vi "UHR-Fleezers Control (host) - Lorentz v4.vi"() -> ()   [LabVIEW 2014] (continued)
            n495 = property on="Green Laser ON" class="Bool (strict)"("Val(Sgnl)"=w901) -> ()  [unwired: 2 in, 2 out]
            n496 = property on="Trap Pos. FB ON" class="Bool (strict)"("Val(Sgnl)"=w901) -> ()  [unwired: 2 in, 2 out]
            n497 = property on="Trap Trig. Fl." class="Bool (strict)"("Val(Sgnl)"=w901) -> ()  [unwired: 2 in, 2 out]
            n498 = property on="Fl. Triggered..." class="Bool (strict)"("Val(Sgnl)"=w901) -> ()  [unwired: 2 in, 2 out]
            n499 = property on="Dip for Protein" class="Bool (strict)"("Val(Sgnl)"=w901) -> ()  [unwired: 2 in, 2 out]
            n500 = property on="Pause dwell" class="Bool (strict)"("Val(Sgnl)"=w901) -> ()  [unwired: 2 in, 2 out]
          }
          frame #2 {
            n501 = property on="Trap Pos. FB Offset Factor" class="DigNum (strict)"("Val(Sgnl)"=i64 0 ("Value (Signaling)")) -> ()  [unwired: 2 in, 2 out]
          }
          frame #3 {
            n502 = local read "Saved Stage Positions"() -> (w910:dbl[][])
            n503 = local write "Stage Moving"(TRUE ("Stage Moving")) -> ()
            n504 = Array Subset(array=w910, index (row)=3 ("index"), length (row)=1 ("length"), index (col)=1 ("index"), length (col)=3 ("length")) -> (w915:dbl[][])
            n505 = Reshape Array(w915, 3 ("dimension size")) -> (w913:dbl[])
            n506 = Array To Cluster(array=w913) -> (cluster=w912:cluster{"[0]":dbl, "[1]":dbl, "[2]":dbl})
            n507 = call "Set Stage Position.vi"("Position"=w912, "error in"=w908, "VISA resource name in"=w909) -> ()  [unwired: 3 out]
          }
          frame #4 {
            w920 = FALSE ("Value (Signaling)")
            n508 = case shown="True" w919 {
              frame False {
              }
              frame True {
                n509 = property on="Sample Channel\nFlow" class="Bool (strict)"("Val(Sgnl)"=FALSE ("Stage Moving")) -> ()  [unwired: 2 in, 2 out]
              }
            }
            n510 = property on="Trap 1 (ON/OFF)" class="Bool (strict)"("Val(Sgnl)"=w920) -> ()  [unwired: 2 in, 2 out]
            n511 = property on="Trap 2 (ON/OFF)" class="Bool (strict)"("Val(Sgnl)"=w920) -> ()  [unwired: 2 in, 2 out]
            n512 = call <vilib>:"Beep.vi"() -> ()  [unwired: 3 in, 9 out]
          }
          frame #5 {
            n513 = property on="Move Cap. 2 (ADig Top)" class="Bool (strict)"("Val(Sgnl)"=TRUE ("Value (Signaling)")) -> ()  [unwired: 2 in, 2 out]
            n514 = property on="Tab Control" class="TabCtl (strict)"("Val(Sgnl)"=T51."Status" ("Value (Signaling)")) -> ()  [unwired: 2 in, 2 out]
          }
        }
      }
      event "Dip for Protein": Value Change {
        n515 = event-data() -> ()  [unwired: 1 in, 5 out]
        n516 = case shown="True" "Dip for Protein" {
          tunnel: w926 -> [_ w928]
          tunnel: w925 -> [_ w927]
          frame False {
          }
          frame True {
            n517 = while {
              tunnel: w928 -> [w939]
              tunnel: w927 -> [w938]
              i -> [w933]
              stop <- w935 stop-if-true
              n518 = Increment(x=w933) -> (x+1=→"Dip #":i32)
              n519 = flat-sequence {
                tunnel: w938 -> [w950]
                tunnel: w939 -> [w951]
                tunnel: [w951] -> w943
                tunnel: [w950] -> w942
                tunnel: [w944] -> w929
                tunnel: [w956] -> w937
                tunnel: [w957] -> w936
                tunnel: w943 -> [w958]
                tunnel: w942 -> [w959]
                tunnel: [w954] -> w930
                tunnel: w929 -> [w954]
                tunnel: [w967] -> w941
                tunnel: w937 -> [w967]
                tunnel: [w966] -> w940
                tunnel: w936 -> [w966]
                tunnel: [w963] -> w934
                tunnel: [w962] -> w931
                tunnel: w930 -> [w962]
                tunnel: w940 -> [w987]
                tunnel: w941 -> [w988]
                tunnel: w934 -> [w989]
                tunnel: w931 -> [w986]
                tunnel: [w1045] -> w935
                frame #0 {
                  n520 = local read "Trap Pos. FB ON"() -> (w944:bool)
                  n521 = Compound Arithmetic op=AND("Flow ON\nduring dip?", "FB OFF when \nflow ON", w944) -> (w945:bool)
                  n522 = case shown="True" "Move trap \nbefore dip move?" {
                    frame False {
                    }
                    frame True {
                      n523 = property on="Trap Delta (MHz)" class="DigNum (strict)"("Val(Sgnl)"="Dipping Delta (MHz)") -> ()  [unwired: 2 in, 2 out]
                    }
                  }
                  n524 = property on="Green Laser ON" class="Bool (strict)"("Val(Sgnl)"="Green ON\nbefore dip?") -> ()  [unwired: 2 in, 2 out]
                  n525 = property on="Sample Channel\nFlow" class="Bool (strict)"("Val(Sgnl)"="Flow ON\nduring dip?") -> ()  [unwired: 2 in, 2 out]
                  n526 = case shown="True" w945 {
                    frame False {
                    }
                    frame True {
                      n527 = property on="Trap Pos. FB ON" class="Bool (strict)"("Val(Sgnl)"=FALSE ("Value (Signaling)")) -> ()  [unwired: 2 in, 2 out]
                    }
                  }
                }
                frame #1 {
                  n528 = local read "Saved Stage Positions"() -> (w961:dbl[][])
                  n529 = local write "Cancel dwell"(FALSE ("Cancel dwell")) -> ()
                  n530 = call "move to saved stage position.vi"("error in"=w959, "Stage VISA resource name in"=w958, "Position"="Dip Stage \nPosition", "Saved Stage Positions"=w961) -> ("VISA resource name out"=w956:refnum<visa-resource-name>, "error out"=w957:errorcluster)
                }
                frame #2 {
                  n531 = node-c288() -> (w965:T35)  [unwired: 4 in]
                  n532 = timed-loop {
                    timing: w965 -> [_]
                    timing-out: [_] -> w964
                    tunnel: [w971] -> w963
                    i -> [w968]
                    stop <- w972 stop-if-true
                    n533 = node-c288() -> ()  [unwired: 1 in, 1 out]
                    n534 = Greater Or Equal?(x=w968, y="Dip Duration (s)") -> (x >= y?=w980:bool)
                    n535 = local read "Dip for Protein"() -> (w973:bool)
                    n536 = local read "Dump Beads"() -> (w970:bool)
                    n537 = local read "Cancel dwell"() -> (w979:bool)
                    n538 = local read "Pause dwell"() -> (w976:bool)
                    n539 = Not(x=w973) -> (.not. x?=w978:bool)
                    n540 = Compound Arithmetic op=OR(w979, w980, w978) -> (w977:bool)
                    n541 = Select(t=FALSE, s=w976, f=w977) -> (s? t:f=w974:bool)
                    n542 = Not(x=w970) -> (.not. x?=w969:bool)
                    n543 = node-c288() -> ()  [unwired: 1 in, 1 out]
                    n544 = And(x=w973, y=w969) -> (x .and. y?=w971:bool)
                    n545 = Or(x=w974, y=w970) -> (x .or. y?=w972:bool)
                    "Dip Time (s)" <- w968
                  }
                  n546 = node-c288(w964) -> ()  [unwired: 1 out]
                }
                frame #3 {
                  n547 = case shown="True" w989 {
                    tunnel: w988 -> [_ w994]
                    tunnel: w987 -> [_ w993]
                    tunnel: w986 -> [_ w990]
                    frame False {
                    }
                    frame True {
                      n548 = flat-sequence {
                        tunnel: w993 -> [w998]
                        tunnel: w994 -> [w999]
                        tunnel: [w999] -> w992
                        tunnel: [w998] -> w991
                        tunnel: w990 -> [w995]
                        tunnel: w992 -> [w1009]
                        tunnel: w991 -> [w1008]
                        tunnel: w990 -> [w1017]
                        frame #0 {
                          n549 = local read "Sample Channel\nFlow"() -> (w997:bool)
                          n550 = case shown="True" w997 {
                            tunnel: "Flow ON \nduring return\nfrom dip?" -> [w1000 w1003]
                            tunnel: w995 -> [_ w1002]
                            frame False {
                              n551 = case shown="True" w1000 {
                                frame False {
                                }
                                frame True {
                                n552 = property on="Sample Channel\nFlow" class="Bool (strict)"("Val(Sgnl)"=TRUE ("Value (Signaling)")) -> ()  [unwired: 2 in, 2 out]
                                }
                              }
                            }
                            frame True {
                              n553 = case shown="False" w1003 {
                                tunnel: w1002 -> [w1004 _]
                                frame False {
                                n554 = property on="Trap Pos. FB ON" class="Bool (strict)"("Val(Sgnl)"=w1004) -> ()  [unwired: 2 in, 2 out]
                                n555 = property on="Sample Channel\nFlow" class="Bool (strict)"("Val(Sgnl)"=FALSE ("Value (Signaling)")) -> ()  [unwired: 2 in, 2 out]
                                }
                                frame True {
                                }
                              }
                            }
                          }
                        }
                        frame #1 {
                          # "For turning on green laser before stage reaches lower spot"
                          n556 = case shown="True" "Green ON\nafter start\nreturn?" {
                            frame False {
                            }
                            frame True {
                              n557 = flat-sequence {
                                frame #0 {
                                n558 = Multiply(x="Green delay after \nstart return (s)", y=1000.0) -> (x*y=w1014:dbl)
                                n559 = Wait (ms)(milliseconds to wait=w1014) -> ()  [unwired: 1 out]
                                }
                                frame #1 {
                                n560 = property on="Green Laser ON" class="Bool (strict)"("Val(Sgnl)"=TRUE ("Value (Signaling)")) -> ()  [unwired: 2 in, 2 out]
                                }
                              }
                            }
                          }
                          n561 = local read "Saved Stage Positions"() -> (w1012:dbl[][])
                          n562 = local write "Cancel dwell"(FALSE ("Cancel dwell")) -> ()
                          n563 = call "move to saved stage position.vi"("error in"=w1008, "Stage VISA resource name in"=w1009, "Position"="Return Stage \nPosition", "Saved Stage Positions"=w1012) -> ("error out"=w1010:errorcluster)  [unwired: 1 out]
                          n564 = local write "Stage Control Serial Error"(w1010) -> ()
                        }
                        frame #2 {
                          n565 = property on="Trap Pos. FB ON" class="Bool (strict)"("Val(Sgnl)"=w1017) -> ()  [unwired: 2 in, 2 out]
                          n566 = case shown="True" "Green ON \nafter return?" {
                            frame False {
                            }
                            frame True {
                              n567 = property on="Green Laser ON" class="Bool (strict)"("Val(Sgnl)"=TRUE ("Value (Signaling)")) -> ()  [unwired: 2 in, 2 out]
                            }
                          }
                          n568 = case shown="True" "Move trap after return?" {
                            frame False {
                            }
                            frame True {
                              n569 = property on="Trap Delta (MHz)" class="DigNum (strict)"("Val(Sgnl)"="Dip Trap Delta 2 (MHz)") -> ()  [unwired: 2 in, 2 out]
                            }
                          }
                          n570 = case shown="True" "Save data after return?" {
                            frame False {
                            }
                            frame True {
                              n571 = property on="Start Saving" class="Bool (strict)"("Val(Sgnl)"=TRUE ("Value (Signaling)")) -> ()  [unwired: 2 in, 2 out]
                            }
                          }
                          n572 = property on="Sample Channel\nFlow" class="Bool (strict)"("Val(Sgnl)"="Flow ON\nduring daq?") -> ()  [unwired: 2 in, 2 out]
                        }
                        frame #3 {
                          n573 = node-c288() -> (w1026:T35)  [unwired: 4 in]
                          n574 = timed-loop {
                            timing: w1026 -> [_]
                            timing-out: [_] -> w1025
                            i -> [w1027]
                            stop <- w1029 stop-if-true
                            n575 = node-c288() -> ()  [unwired: 1 in, 1 out]
                            n576 = local read "Dump Beads"() -> (w1028:bool)
                            n577 = Greater Or Equal?(x=w1027, y="Dwell Duration (s)") -> (x >= y?=w1034:bool)
                            n578 = local read "Dip for Protein"() -> (w1031:bool)
                            n579 = Not(x=w1031) -> (.not. x?=w1030:bool)
                            n580 = Compound Arithmetic op=OR(w1034, "Cancel dwell", w1030) -> (w1033:bool)
                            n581 = node-c288() -> ()  [unwired: 1 in, 1 out]
                            n582 = Select(t=FALSE, s="Pause dwell", f=w1033) -> (s? t:f=w1036:bool)
                            n583 = Or(x=w1036, y=w1028) -> (x .or. y?=w1029:bool)
                            "Dwell Time (s)" <- w1027
                          }
                          n584 = node-c288(w1025) -> ()  [unwired: 1 out]
                        }
                      }
                    }
                  }
                }
                frame #4 {
                  n585 = local read "Dip for Protein"() -> (w1046:bool)
                  n586 = local read "Dump Beads"() -> (w1043:bool)
                  n587 = local write "Cancel dwell"(FALSE ("Cancel dwell")) -> ()
                  n588 = Not(x=w1046) -> (.not. x?=w1047:bool)
                  n589 = Not(x="Cont. Repeat Dipping?") -> (.not. x?=w1049:bool)
                  n590 = Compound Arithmetic op=OR(w1047, w1049, w1043) -> (w1045:bool)
                }
              }
            }
          }
        }
      }
      event "Profile": Value Change {
        n591 = event-data() -> ()  [unwired: 1 in, 5 out]
        n592 = flat-sequence {
          tunnel: w1058 -> [w1061]
          tunnel: w1057 -> [w1069]
          tunnel: [w1063] -> w1056
          tunnel: [w1062] -> w1055
          tunnel: [w1060] -> w1053
          tunnel: [w1059] -> w1050
          tunnel: w1056 -> [w1076]
          tunnel: w1055 -> [w1075]
          tunnel: [w1073] -> w1054
          tunnel: w1053 -> [w1074]
          tunnel: [w1072] -> w1052
          tunnel: [w1071] -> w1051
          tunnel: w1050 -> [w1071]
          tunnel: w1054 -> [w1080]
          tunnel: w1052 -> [w1079]
          tunnel: w1051 -> [w1078]
          frame #0 {
            n593 = call "Read Stage Position.vi"("error in"=w1069, "VISA resource name in"=w1061) -> ("Current Position"=w1059:cluster{dbl, dbl, dbl}, "error out"=w1062:errorcluster, "VISA resource name out"=w1060:refnum<visa-resource-name>)  [unwired: 1 out]
            "Current Position" <- w1059
            n594 = local write "Stage Control Serial Error"(w1062) -> ()
            n595 = Unbundle(w1059) -> (w1066:dbl, w1068:dbl, w1064:dbl)
            n596 = Add(x=w1068, y="Y change (mm)") -> (x+y=w1065:dbl)
            n597 = Bundle(w1066, w1065, w1064) -> (w1063:cluster{dbl, dbl, dbl})  [unwired: 1 in]
          }
          frame #1 {
            # "move to new position and start saving"
            n598 = local write "Stage Moving"(TRUE ("Stage Moving")) -> ()
            n599 = local write "Start Saving"(TRUE ("Start Saving")) -> ()
            n600 = call "Set Stage Position.vi"("Position"=w1076, "error in"=w1075, "VISA resource name in"=w1074) -> ("error out"=w1072:errorcluster, "VISA resource name out"=w1073:refnum<visa-resource-name>)  [unwired: 1 out]
          }
          frame #2 {
            # "go back to start"
            n601 = call "Set Stage Position.vi"("Position"=w1078, "error in"=w1079, "VISA resource name in"=w1080) -> ()  [unwired: 3 out]
          }
          frame #3 {
            # "stop saving"
            n602 = local write "Stop Saving"(TRUE ("Stop Saving")) -> ()
            n603 = local write "Stage Moving"(FALSE ("Stage Moving")) -> ()
          }
        }
      }
      event "Move to Position 1", "Move to Position 2", "Move to Position 3", "Move to Position 4", "Move to Position 5", "Lower Ch. Cap.", "Move to Position 6": Value Change {
        n604 = event-data() -> ()  [unwired: 1 in, 5 out]
        n605 = Or(x="Move to Position 5", y="Lower Ch. Cap.") -> (x .or. y?=w1087:bool)
        n606 = Build Array("Move to Position 1", "Move to Position 2", "Move to Position 3", "Move to Position 4", w1087, "Move to Position 6") -> (w1090:bool[])
        n607 = Boolean Array To Number(Boolean array=w1090) -> (number=w1089:u32)
        n608 = Logarithm Base 2(1:w1089) -> (0:w1088:dbl)
        n609 = flat-sequence {
          tunnel: w1088 -> [w1099]
          tunnel: w1085 -> [w1097]
          tunnel: w1084 -> [w1096]
          frame #0 {
            n610 = local read "Saved Stage Positions"() -> (w1107:dbl[][])
            n611 = Array Subset(array=w1107, index (row)=w1099, length (row)=1 ("length"), index (col)=1 ("index"), length (col)=3 ("length")) -> (w1104:dbl[][])
            n612 = Reshape Array(w1104, 3 ("dimension size")) -> (w1102:dbl[])
            n613 = Array To Cluster(array=w1102) -> (cluster=w1101:cluster{"[0]":dbl, "[1]":dbl, "[2]":dbl})
            n614 = call "Set Stage Position.vi"("Position"=w1101, "error in"=w1096, "VISA resource name in"=w1097) -> ("error out"=w1100:errorcluster)  [unwired: 2 out]
            n615 = local write "Stage Moving"(TRUE ("Stage Moving")) -> ()
            n616 = local write "Stage Control Serial Error"(w1100) -> ()
          }
          frame #1 {
            n617 = local write "Stage Moving"(FALSE ("Stage Moving")) -> ()
            n618 = call <vilib>:"Beep.vi"() -> ()  [unwired: 3 in, 9 out]
          }
        }
      }
      event "Got Bead 1": Value Change {
        n619 = event-data() -> ()  [unwired: 1 in, 5 out]
        n620 = flat-sequence {
          tunnel: w1110 -> [w1112]
          tunnel: w1110 -> [w1116]
          frame #0 {
            n621 = for {
              N: w1112 -> [_]
              n622 = property on="Pressure Up" class="Bool (strict)"("Val(Sgnl)"=TRUE) -> ()  [unwired: 2 in, 2 out]
            }
          }
          frame #1 {
          }
          frame #2 {
            n623 = Wait (ms)(milliseconds to wait=u32 1000) -> ()  [unwired: 1 out]
          }
          frame #3 {
          }
          frame #4 {
            n624 = Multiply(x=w1116, y=2) -> (x*y=w1115:i32)
            n625 = for {
              N: w1115 -> [_]
              n626 = property on="Vent pressure" class="Bool (strict)"("Val(Sgnl)"=TRUE) -> ()  [unwired: 2 in, 2 out]
            }
          }
          frame #5 {
            n627 = for {
              N: "Number of Pulses for bead 2" -> [_]
              n628 = property on="Pressure Up" class="Bool (strict)"("Val(Sgnl)"=TRUE) -> ()  [unwired: 2 in, 2 out]
            }
          }
        }
        n629 = local read "Number of pulses For laminar flow"() -> (w1110:i32)
      }
      event "Force FB Data\nScript": Value Change {
        n630 = event-data() -> ()  [unwired: 1 in, 5 out]
        n631 = flat-sequence {
          tunnel: w1126 -> [w1130]
          tunnel: w1127 -> [w1131]
          tunnel: [w1131] -> w1122
          tunnel: [w1130] -> w1121
          tunnel: w1122 -> [w1134]
          tunnel: w1121 -> [w1133]
          tunnel: ["Trap Trig Fl."] -> w1123
          tunnel: [w1159] -> w1124
          tunnel: w1123 -> [w1159]
          tunnel: [w1163] -> w1125
          tunnel: w1124 -> [w1163]
          tunnel: w1125 -> [w1165]
          frame #0 {
            n632 = property on="Trap Delta (MHz)" class="DigNum (strict)"("Val(Sgnl)"="Trap Delta Before Moving") -> ()  [unwired: 2 in, 2 out]
          }
          frame #1 {
            n633 = local read "Saved Stage Positions"() -> (w1136:dbl[][])
            n634 = property on="Trap Pos. FB Offset Factor" class="DigNum (strict)"("Val(Sgnl)"=i64 0 ("Value (Signaling)")) -> ()  [unwired: 2 in, 2 out]
            n635 = local write "FB Trap Pos Offset"(0.0 ("FB Trap Pos Offset")) -> ()
            n636 = local write "Stage Moving"(TRUE ("Stage Moving")) -> ()
            n637 = call "move to saved stage position.vi"("error in"=w1133, "Stage VISA resource name in"=w1134, "Position"="Stage Position To Establish FB", "Saved Stage Positions"=w1136) -> ("error out"=w1132:errorcluster)  [unwired: 1 out]
            n638 = local write "Stage Control Serial Error"(w1132) -> ()
          }
          frame #2 {
            n639 = call <vilib>:"Beep.vi"() -> ()  [unwired: 3 in, 9 out]
            n640 = Multiply(x="Wait (s)", y=u32 1000 ("milliseconds to wait")) -> (x*y=w1143:u32)
            n641 = property on="Trap Delta (MHz)" class="DigNum (strict)"("Val(Sgnl)"="Starting \nTrap Delta (MHz)") -> ()  [unwired: 2 in, 2 out]
            n642 = local write "Stage Moving"(FALSE ("Stage Moving")) -> ()
            n643 = Wait (ms)(milliseconds to wait=w1143) -> ()  [unwired: 1 out]
            n644 = property on="Tab Control 2" class="TabCtl (strict)"("Val(Sgnl)"=T11."Feedback on Trap Position" ("Value (Signaling)")) -> ()  [unwired: 2 in, 2 out]
            n645 = property on="Tab Control" class="TabCtl (strict)"("Val(Sgnl)"=T52."Trap Control (RF)" ("Value (Signaling)")) -> ()  [unwired: 2 in, 2 out]
          }
          frame #3 {
            n646 = property on="Set Reading to\nSetpoint" class="Bool (strict)"("Val(Sgnl)"=TRUE ("Value (Signaling)")) -> ()  [unwired: 2 in, 2 out]
            n647 = Wait (ms)(milliseconds to wait=u32 500) -> ()  [unwired: 1 out]
          }
          frame #4 {
            n648 = property on="Trap Pos. FB ON" class="Bool (strict)"("Val(Sgnl)"=TRUE ("Value (Signaling)")) -> ()  [unwired: 2 in, 2 out]
            n649 = Wait (ms)(milliseconds to wait=u32 250) -> ()  [unwired: 1 out]
          }
          frame #5 {
            n650 = case shown="False" "Trap Trig Fl." {
              frame False {
                n651 = case shown="True" "Green ON after FB ON?" {
                  selector: "Green ON after FB ON?" -> [_ w1158]
                  frame False {
                  }
                  frame True {
                    n652 = property on="Green Laser ON" class="Bool (strict)"("Val(Sgnl)"=w1158) -> ()  [unwired: 2 in, 2 out]
                  }
                }
              }
              frame True {
              }
            }
            n653 = case shown="True" "Remove Action Offset" {
              tunnel: TRUE ("Value (Signaling)") -> [w1155 w1156]
              frame False {
                n654 = property on="Remove Unwinding Offset" class="Bool (strict)"("Val(Sgnl)"=w1155) -> ()  [unwired: 2 in, 2 out]
              }
              frame True {
                n655 = property on="Remove Action Offset" class="Bool (strict)"("Val(Sgnl)"=w1156) -> ()  [unwired: 2 in, 2 out]
              }
            }
            n656 = Wait (ms)(milliseconds to wait=u32 250) -> ()  [unwired: 1 out]
          }
          frame #6 {
            n657 = property on="Start Saving" class="Bool (strict)"("Val(Sgnl)"=TRUE ("Value (Signaling)")) -> ()  [unwired: 2 in, 2 out]
            n658 = Wait (ms)(milliseconds to wait=u32 5000) -> ()  [unwired: 1 out]
          }
          frame #7 {
            w1162 = TRUE ("Value (Signaling)")
            n659 = property on="Rem fb disp offset" class="Bool (strict)"("Val(Sgnl)"=w1162) -> ()  [unwired: 2 in, 2 out]
            n660 = property on="Remove Offset" class="Bool (strict)"("Val(Sgnl)"=w1162) -> ()  [unwired: 2 in, 2 out]
            n661 = Wait (ms)(milliseconds to wait=u32 100) -> ()  [unwired: 1 out]
          }
          frame #8 {
            n662 = case shown="True" w1165 {
              frame False {
              }
              frame True {
                n663 = local write "Trap Trig. Fl."(TRUE ("Value (Signaling)")) -> ()
              }
            }
          }
          frame #9 {
            n664 = case shown="True" "Start dipping after?" {
              frame False {
              }
              frame True {
                n665 = flat-sequence {
                  frame #0 {
                    n666 = Multiply(x="Delay before dipping (s)", y=1000.0) -> (x*y=w1169:dbl)
                    n667 = Wait (ms)(milliseconds to wait=w1169) -> ()  [unwired: 1 out]
                  }
                  frame #1 {
                    n668 = property on="Dip for Protein" class="Bool (strict)"("Val(Sgnl)"=TRUE ("Value (Signaling)")) -> ()  [unwired: 2 in, 2 out]
                    n669 = local write "Scripts"(T3."Dipping" ("Scripts")) -> ()
                  }
                }
              }
            }
          }
        }
      }
      event "Fixed Traps Data\nScript": Value Change {
        n670 = event-data() -> ()  [unwired: 1 in, 5 out]
        n671 = flat-sequence {
          frame #0 {
            n672 = case shown="True" "Green ON" {
              frame False {
              }
              frame True {
                n673 = property on="Green Laser ON" class="Bool (strict)"("Val(Sgnl)"=TRUE) -> ()  [unwired: 2 in, 2 out]
              }
            }
            n674 = local write "Offset (nm)"(0.0 ("Offset (nm)")) -> ()
            n675 = property on="Sample Channel\nFlow" class="Bool (strict)"("Val(Sgnl)"=FALSE ("Value (Signaling)")) -> ()  [unwired: 2 in, 2 out]
            n676 = property on="Trap Delta (MHz)" class="DigNum (strict)"("Val(Sgnl)"="Fixed Traps Trap Delta (MHz)") -> ()  [unwired: 2 in, 2 out]
          }
          frame #1 {
            n677 = Wait (ms)(milliseconds to wait=u32 1000) -> ()  [unwired: 1 out]
          }
          frame #2 {
            n678 = local write "Start Saving"(TRUE ("Start Saving")) -> ()
          }
          frame #3 {
            n679 = local read "Bead Sep. Int. Time (s)"() -> (w1180:dbl)
            n680 = Multiply(x=w1180, y=1000.0) -> (x*y=w1182:dbl)
            n681 = Wait (ms)(milliseconds to wait=w1182) -> ()  [unwired: 1 out]
          }
          frame #4 {
            n682 = property on="Remove Offset" class="Bool (strict)"("Val(Sgnl)"=TRUE ("Value (Signaling)")) -> ()  [unwired: 2 in, 2 out]
          }
          frame #5 {
            n683 = property on="Dip for Protein" class="Bool (strict)"("Val(Sgnl)"="Start dipping after?") -> ()  [unwired: 2 in, 2 out]
          }
        }
      }
      event "Got Bead 2": Value Change {
        # "Got A Dig bead and Got DNA bead events changes by Ronen to Got bead 1 and Got bead 2, and modified to enable operation of the thorlabs motors."
        n684 = event-data() -> ()  [unwired: 1 in, 5 out]
        n685 = flat-sequence {
          tunnel: w1185 -> [w1188]
          frame #0 {
            n686 = case shown="True" "Lumicks Flow During Calibration" {
              tunnel: w1188 -> [_ w1189]
              frame False {
              }
              frame True {
                n687 = for {
                  N: w1189 -> [_]
                  n688 = property on="Pressure Up" class="Bool (strict)"("Val(Sgnl)"=TRUE) -> ()  [unwired: 2 in, 2 out]
                }
              }
            }
          }
          frame #1 {
          }
          frame #2 {
            n689 = Wait (ms)(milliseconds to wait=u32 1000) -> ()  [unwired: 1 out]
          }
          frame #3 {
          }
          frame #4 {
            n690 = case shown="True" "Calibrate after bead 2?" {
              frame False {
              }
              frame True {
                n691 = property on="Cal/Data Acq. Spot" class="Bool (strict)"("Val(Sgnl)"=TRUE) -> ()  [unwired: 2 in, 2 out]
              }
            }
          }
        }
        n692 = local read "Number of pulses For laminar flow"() -> (w1185:i32)
      }
      event "Get New Beads": Value Change {
        # "Flow Control determines how many pressure increases are given when moving."
        n693 = event-data() -> ()  [unwired: 1 in, 6 out]
        n694 = flat-sequence {
          tunnel: w1194 -> [w1196]
          tunnel: w1194 -> [w1200]
          frame #0 {
            n695 = for {
              N: w1196 -> [_]
              n696 = property on="Pressure Up" class="Bool (strict)"("Val(Sgnl)"=TRUE) -> ()  [unwired: 2 in, 2 out]
            }
          }
          frame #1 {
          }
          frame #2 {
            n697 = Wait (ms)(milliseconds to wait=u32 1000) -> ()  [unwired: 1 out]
          }
          frame #3 {
          }
          frame #4 {
            n698 = Multiply(x=2, y=w1200) -> (x*y=w1199:i32)
            n699 = for {
              N: w1199 -> [_]
              n700 = property on="Vent pressure" class="Bool (strict)"("Val(Sgnl)"=TRUE) -> ()  [unwired: 2 in, 2 out]
            }
          }
          frame #5 {
            n701 = for {
              N: "Number of pulses for Bead 1" -> [_]
              n702 = property on="Pressure Up" class="Bool (strict)"("Val(Sgnl)"=TRUE) -> ()  [unwired: 2 in, 2 out]
            }
          }
        }
        n703 = local read "Number of pulses For laminar flow"() -> (w1194:i32)
      }
      event "Take Stepping Data": Value Change {
        n704 = event-data() -> ()  [unwired: 1 in, 5 out]
        n705 = local read "Save ave N"() -> (w1213:dbl)
        n706 = flat-sequence {
          tunnel: w1213 -> [w1215]
          tunnel: [w1215] -> w1208
          tunnel: [w1217] -> w1209
          tunnel: w1208 -> [w1217]
          tunnel: [w1219] -> w1210
          tunnel: w1209 -> [w1219]
          tunnel: [w1222] -> w1211
          tunnel: w1210 -> [w1222]
          tunnel: [w1224] -> w1212
          tunnel: w1211 -> [w1224]
          tunnel: [w1226] -> w1206
          tunnel: w1212 -> [w1226]
          tunnel: w1206 -> [w1229]
          tunnel: [w1229] -> w1205
          tunnel: w1205 -> [w1230]
          tunnel: [w1230] -> w1207
          tunnel: w1207 -> [w1236]
          frame #0 {
            n707 = property on="Save ave N" class="DigNum (strict)"("Val(Sgnl)"="Save ave factor") -> ()  [unwired: 2 in, 2 out]
          }
          frame #1 {
            n708 = Wait (ms)(milliseconds to wait=u32 100) -> ()  [unwired: 1 out]
          }
          frame #2 {
            n709 = local read "Offset 2 Start (MHz)"() -> (w1221:dbl)
            n710 = property on="Saved AOD Raster Scan Parameter Sets" class="Arr (strict)"("Index Values"=u32[] [2]) -> ()  [unwired: 2 in, 2 out]
            n711 = property on="Trap Delta (MHz)" class="DigNum (strict)"("Val(Sgnl)"=w1221) -> ()  [unwired: 2 in, 2 out]
          }
          frame #3 {
            n712 = property on="Load parameters" class="Bool (strict)"("Val(Sgnl)"=TRUE ("Value (Signaling)")) -> ()  [unwired: 2 in, 2 out]
          }
          frame #4 {
            n713 = Wait (ms)(milliseconds to wait=u32 100) -> ()  [unwired: 1 out]
          }
          frame #5 {
            n714 = property on="Trap Raster Scan" class="Bool (strict)"("Val(Sgnl)"=TRUE ("Value (Signaling)")) -> ()  [unwired: 2 in, 2 out]
          }
          frame #6 {
            n715 = Wait (ms)(milliseconds to wait=u32 1000) -> ()  [unwired: 1 out]
          }
          frame #7 {
            n716 = while {
              stop <- w1233 stop-if-true
              n717 = local read "Raster Scanning..."() -> (w1235:bool)
              n718 = local read "Saving..."() -> (w1234:bool)
              n719 = Not(x=w1234) -> (.not. x?=w1231:bool)
              n720 = Not(x=w1235) -> (.not. x?=w1232:bool)
              n721 = And(x=w1232, y=w1231) -> (x .and. y?=w1233:bool)
            }
          }
          frame #8 {
            n722 = property on="Save ave N" class="DigNum (strict)"("Val(Sgnl)"=w1236) -> ()  [unwired: 2 in, 2 out]
          }
        }
      }
      event "Step Size (nm)": Value Change {
        n723 = event-data() -> ()  [unwired: 1 in, 5 out]
        n724 = flat-sequence {
          frame #0 {
            n725 = property on="Saved AOD Raster Scan Parameter Sets" class="Arr (strict)"("Index Values"=u32[] [1]) -> ()  [unwired: 2 in, 2 out]
          }
          frame #1 {
            n726 = Multiply(x="N Steps", y="Step Size (nm)") -> (x*y=w1238:dbl)
            n727 = property on="Scan Speed AOD (nm/s) 2" class="DigNum (strict)"("Value"="Step Size (nm)") -> ()  [unwired: 2 in, 2 out]
            n728 = property on="Step Size AOD (nm) 2" class="DigNum (strict)"("Value"="Step Size (nm)") -> ()  [unwired: 2 in, 2 out]
            n729 = property on="Scan Range AOD (nm) 2" class="DigNum (strict)"("Value"=w1238) -> ()  [unwired: 2 in, 2 out]
          }
        }
      }
      event "Take Detection Laser\nImage": Value Change {
        n730 = event-data() -> ()  [unwired: 1 in, 5 out]
        n731 = flat-sequence {
          tunnel: [w1266] -> w1256
          tunnel: [w1265] -> w1249
          tunnel: [w1264] -> w1241
          tunnel: [w1269] -> w1257
          tunnel: w1256 -> [w1269]
          tunnel: [w1268] -> w1250
          tunnel: w1249 -> [w1268]
          tunnel: [w1267] -> w1242
          tunnel: w1241 -> [w1267]
          tunnel: [w1273] -> w1258
          tunnel: w1257 -> [w1273]
          tunnel: [w1272] -> w1251
          tunnel: w1250 -> [w1272]
          tunnel: [w1271] -> w1243
          tunnel: w1242 -> [w1271]
          tunnel: [w1279] -> w1259
          tunnel: w1258 -> [w1279]
          tunnel: [w1278] -> w1252
          tunnel: w1251 -> [w1278]
          tunnel: [w1277] -> w1244
          tunnel: w1243 -> [w1277]
          tunnel: [w1283] -> w1260
          tunnel: w1259 -> [w1283]
          tunnel: [w1282] -> w1253
          tunnel: w1252 -> [w1282]
          tunnel: [w1281] -> w1245
          tunnel: w1244 -> [w1281]
          tunnel: [w1287] -> w1261
          tunnel: w1260 -> [w1287]
          tunnel: [w1286] -> w1254
          tunnel: w1253 -> [w1286]
          tunnel: [w1285] -> w1246
          tunnel: w1245 -> [w1285]
          tunnel: [w1291] -> w1262
          tunnel: w1261 -> [w1291]
          tunnel: [w1290] -> w1255
          tunnel: w1254 -> [w1290]
          tunnel: [w1289] -> w1247
          tunnel: w1246 -> [w1289]
          tunnel: w1262 -> [w1297]
          tunnel: w1255 -> [w1296]
          tunnel: [w1294] -> w1248
          tunnel: w1247 -> [w1294]
          tunnel: w1248 -> [w1298]
          frame #0 {
            n732 = local read "Laser interlacing mode"() -> (w1265:enum32{"Laser ON", "Laser OFF", "Interlace"})
            n733 = local read "Green FB On/Off"() -> (w1264:bool)
            n734 = local read "Green Laser ON"() -> (w1266:bool)
          }
          frame #1 {
            n735 = property on="Green FB On/Off" class="Bool (strict)"("Val(Sgnl)"=FALSE ("Value (Signaling)")) -> ()  [unwired: 2 in, 2 out]
          }
          frame #2 {
            n736 = property on="Green Laser ON" class="Bool (strict)"("Val(Sgnl)"=TRUE ("Value (Signaling)")) -> ()  [unwired: 2 in, 2 out]
            n737 = property on="Flip Green Filter" class="Bool (strict)"("Val(Sgnl)"=TRUE ("Value (Signaling)")) -> ()  [unwired: 2 in, 2 out]
            n738 = property on="Laser interlacing mode" class="RadioBtnsControl (strict)"("Val(Sgnl)"=enum32{"Laser ON", "Laser OFF", "Interlace"}."Laser ON" ("Value (Signaling)")) -> ()  [unwired: 2 in, 2 out]
          }
          frame #3 {
            n739 = Wait (ms)(milliseconds to wait=u32 500) -> ()  [unwired: 1 out]
          }
          frame #4 {
            n740 = property on="Confocal Image" class="Bool (strict)"("Val(Sgnl)"=TRUE ("Value (Signaling)")) -> ()  [unwired: 2 in, 2 out]
          }
          frame #5 {
            n741 = Wait (ms)(milliseconds to wait=u32 2000) -> ()  [unwired: 1 out]
          }
          frame #6 {
            n742 = while {
              stop <- w1292 stop-if-true
              n743 = local read "Saving..."() -> (w1293:bool)
              n744 = Not(x=w1293) -> (.not. x?=w1292:bool)
            }
          }
          frame #7 {
            n745 = property on="Flip Green Filter" class="Bool (strict)"("Val(Sgnl)"=TRUE ("Value (Signaling)")) -> ()  [unwired: 2 in, 2 out]
            n746 = property on="Green Laser ON" class="Bool (strict)"("Val(Sgnl)"=w1297) -> ()  [unwired: 2 in, 2 out]
            n747 = property on="Laser interlacing mode" class="RadioBtnsControl (strict)"("Val(Sgnl)"=w1296) -> ()  [unwired: 2 in, 2 out]
          }
          frame #8 {
            n748 = property on="Green FB On/Off" class="Bool (strict)"("Val(Sgnl)"=w1298) -> ()  [unwired: 2 in, 2 out]
          }
        }
      }
      event "Move in a Circle": Value Change {
        w1300 = dbl[] []
        # "converting distance (d) to angle (a)\na=arcsin(d/2r)"
        # "radius"
        # "radius"
        # "T1 Y"
        # "T1 X"
        n749 = event-data() -> ()  [unwired: 1 in, 5 out]
        n750 = local read "BD 1 Frequency 1 (MHz)"() -> (w1308:dbl)
        n751 = local read "BD 2 Frequency 1 (MHz)"() -> (w1307:dbl)
        n752 = local read "BD 1 Frequency 2 (MHz)"() -> (w1306:dbl)
        n753 = local read "BD 2 Frequency 2 (MHz)"() -> (w1305:dbl)
        n754 = Subtract(x=w1307, y="Center Y Frequency (MHz)") -> (x-y=w1312:dbl)
        n755 = Absolute Value(x=w1312) -> (abs(x)=w1303:dbl)
        n756 = flat-sequence {
          tunnel: w1303 -> [w1315]
          tunnel: [w1315] -> w1302
          frame #0 {
            n757 = local write "Radius (MHz)"(w1315) -> ()
          }
        }
        n758 = node-c288("Time step (ms)") -> (w1314:T35)  [unwired: 3 in]
        n759 = timed-loop {
          timing: w1314 -> [_]
          timing-out: [_] -> w1313
          tunnel: w1308 -> [w1406]
          tunnel: w1307 -> [_]
          tunnel: w1306 -> [w1410]
          tunnel: w1305 -> [_]
          tunnel: "Center Y Frequency (MHz)" -> [w1399]
          shift-right: [w1360] -> _
          shift-left: w1300 -> [w1367]
          shift-right: [w1358] -> _
          shift-left: w1300 -> [w1366]
          shift-right: [w1351] -> _
          shift-left: w1300 -> [w1364]
          shift-right: [w1349] -> _
          shift-left: w1300 -> [w1363]
          tunnel: "Move in a Circle" -> [_]
          tunnel: ["Back to start on finish?"] -> w1304
          tunnel: w1302 -> [_]
          tunnel: w1301 -> [w1381]
          tunnel: w1300 -> [w1362]
          shift-right: [w1333] -> _
          shift-left: 0.0 -> [w1331]
          i -> [w1340]
          stop <- w1404 stop-if-true
          w1348 = 0 ("index")
          w1369 = 1 ("dimension size")
          # "Keep phase within\n2pi so errors don't \nbuild"
          # "Accumulated\nphase"
          # "Current phase"
          # "Trap 2"
          # "Trap 1"
          # "ignore if N = 0"
          # "r"
          # "r"
          # "r"
          # "r"
          # "\"omega*t\""
          # "Trap 2"
          # "Trap separation (radians)"
          # "Trap 1"
          # "Offset (starts\n at bottom of\n the circle)"
          # "omega"
          n760 = node-c288() -> (w1417:i64)  [unwired: 1 in]
          n761 = Divide(x=w1417, y=1000) -> (x/y=w1336:dbl)
          n762 = Divide(x="2D Motion Trap Separation (MHz)", y="Radius (MHz)") -> (x/y=w1391:dbl)
          n763 = Negate(x=w1336) -> (-x=w1335:dbl)
          n764 = Divide(x="Trap 2 phase shift (deg)", y=360.0) -> (x/y=w1382:dbl)
          n765 = Inverse Sine(1:w1391) -> (0:w1327:dbl)
          n766 = Multiply(x=6.283185307179586, y=w1382) -> (x*y=w1328:dbl)
          n767 = Multiply(x=6.283185307179586, y="2D Motion Frequency (Hz)") -> (x*y=w1339:dbl)
          n768 = Select(t=w1336, s="Counterclockwise/Clockwise", f=w1335) -> (s? t:f=w1338:dbl)
          n769 = Multiply(x=w1339, y=w1338) -> (x*y=w1329:dbl)
          n770 = Select(t=w1327, s="Trap shift\nmethod", f=w1328) -> (s? t:f=w1326:dbl)
          n771 = Add(x=w1329, y=w1331) -> (x+y=w1332:dbl)
          n772 = Add(x=w1332, y=w1326) -> (x+y=w1388:dbl)
          n773 = Add(x=w1332, y=1.5707963267948966) -> (x+y=w1337:dbl)
          n774 = Add(x=w1388, y=1.5707963267948966) -> (x+y=w1401:dbl)
          n775 = Cosine(x=w1337) -> (cos(x)=w1415:dbl)
          n776 = Sine(x=w1337) -> (sin(x)=w1414:dbl)
          n777 = Multiply(x=w1415, y="Radius (MHz)") -> (x*y=w1408:dbl)
          n778 = Cosine(x=w1401) -> (cos(x)=w1413:dbl)
          n779 = Sine(x=w1401) -> (sin(x)=w1412:dbl)
          n780 = Multiply(x=w1414, y="Radius (MHz)") -> (x*y=w1407:dbl)
          n781 = Multiply(x=w1413, y="Radius (MHz)") -> (x*y=w1411:dbl)
          n782 = Multiply(x=w1412, y="Radius (MHz)") -> (x*y=w1409:dbl)
          n783 = Add(x=w1408, y=w1406) -> (x+y=w1357:dbl)
          n784 = Add(x=w1407, y=w1399) -> (x+y=w1355:dbl)
          n785 = Greater Or Equal?(x=w1340, y="N steps then stop") -> (x >= y?=w1398:bool)
          n786 = Add(x=w1411, y=w1410) -> (x+y=w1346:dbl)
          n787 = Add(x=w1409, y=w1399) -> (x+y=w1344:dbl)
          n788 = Not Equal To 0?(x="N steps then stop") -> (x != 0?=w1394:bool)
          n789 = And(x=w1398, y=w1394) -> (x .and. y?=w1395:bool)
          n790 = local read "Trap 1 sum mean"() -> (w1378:dbl)
          n791 = local read "Stop All"() -> (w1403:bool)
          n792 = local write "BD 1 Frequency 1 (MHz)"(w1357) -> ()
          n793 = local write "BD 2 Frequency 1 (MHz)"(w1355) -> ()
          n794 = local write "BD 1 Frequency 2 (MHz)"(w1346) -> ()
          n795 = local write "BD 2 Frequency 2 (MHz)"(w1344) -> ()
          n796 = Select(t=w1340, s="test", f=w1378) -> (s? t:f=→"Waveform Chart":dbl)
          n797 = Compound Arithmetic op=OR(w1403, "Stop Moving", w1395) -> (w1404:bool)
          n798 = local read "BD 1 Frequency 3 (MHz)"() -> (w1387:dbl)
          n799 = local read "BD 2 Frequency 3 (MHz)"() -> (w1386:dbl)
          n800 = Select(t=w1362, s="Reset graph", f=w1363) -> (s? t:f=w1343:dbl[])
          n801 = Select(t=w1362, s="Reset graph", f=w1364) -> (s? t:f=w1345:dbl[])
          n802 = Select(t=w1362, s="Reset graph", f=w1366) -> (s? t:f=w1354:dbl[])
          n803 = Select(t=w1362, s="Reset graph", f=w1367) -> (s? t:f=w1356:dbl[])
          n804 = Initialize Array(w1344, w1369) -> (w1370:dbl[])
          n805 = Initialize Array(w1355, w1369) -> (w1373:dbl[])
          n806 = Initialize Array(w1346, w1369) -> (w1371:dbl[])
          n807 = Initialize Array(w1357, w1369) -> (w1374:dbl[])
          n808 = local read "Y RF Frequency Limits (MHz)"() -> (w1384:T24)
          n809 = local read "X RF Frequency Limits (MHz)"() -> (w1385:T24)
          n810 = call "set RF board frequency - interlace.vi"("Board 2 Frequency Limits"=w1384, "Board 1 Frequency Limits"=w1385, "FPGA VI Reference In"=w1381, "Board 2 Frequency 3 (MHz)"=w1386, "Board 1 Frequency 3 (MHz)"=w1387, "Board 2 Frequency 2 (MHz)"=w1344, "Board 2 Frequency 1 (MHz)"=w1355, "Board 1 Frequency 2 (MHz)"=w1346, "Board 1 Frequency 1  (MHz)"=w1357) -> ()  [unwired: 1 in, 2 out]
          n811 = Bundle(w1371, w1370) -> (w1342:cluster{dbl[], dbl[]})  [unwired: 1 in]
          n812 = Bundle(w1374, w1373) -> (w1372:cluster{dbl[], dbl[]})  [unwired: 1 in]
          n813 = Build Array (concatenate)(w1357, w1356) -> (w1361:dbl[])
          n814 = Build Array (concatenate)(w1355, w1354) -> (w1359:dbl[])
          n815 = Build Array (concatenate)(w1346, w1345) -> (w1352:dbl[])
          n816 = Build Array (concatenate)(w1344, w1343) -> (w1350:dbl[])
          n817 = Bundle(w1361, w1359) -> (w1341:cluster{dbl[], dbl[]})  [unwired: 1 in]
          n818 = Bundle(w1352, w1350) -> (w1368:cluster{dbl[], dbl[]})  [unwired: 1 in]
          n819 = Build Array(w1372, w1342, w1341, w1368) -> (→"Trap trajectories":cluster{dbl[], dbl[]}[])
          n820 = case "To pause the process" shown="True" "Pause rotation" {
            frame False {
            }
            frame True {
              n821 = while {
                stop <- w1420 stop-if-true
                n822 = local read "Pause rotation"() -> (w1421:bool)
                n823 = Wait (ms)(milliseconds to wait=u32 10) -> ()  [unwired: 1 out]
                n824 = Not(x=w1421) -> (.not. x?=w1420:bool)
              }
            }
          }
          n825 = Decrement(x="N steps to plot") -> (x-1=w1347:i32)
          n826 = Array Subset(array=w1359, index=w1348, length=w1347) -> (w1358:dbl[])
          n827 = Array Subset(array=w1361, index=w1348, length=w1347) -> (w1360:dbl[])
          n828 = Array Subset(array=w1352, index=w1348, length=w1347) -> (w1351:dbl[])
          n829 = Array Subset(array=w1350, index=w1348, length=w1347) -> (w1349:dbl[])
          n830 = Quotient & Remainder(x=w1332, y=6.283185307179586) -> (x-y*floor(x/y)=w1333:dbl)  [unwired: 1 out]
          n831 = node-c288() -> ()  [unwired: 1 in, 1 out]
        }
        n832 = node-c288(w1313) -> ()  [unwired: 1 out]
        n833 = case shown="True" w1304 {
          tunnel: w1308 -> [_ w1319]
          tunnel: w1307 -> [_ w1318]
          tunnel: w1306 -> [_ w1317]
          tunnel: w1305 -> [_ w1316]
          frame False {
          }
          frame True {
            n834 = flat-sequence {
              tunnel: w1319 -> [w1323]
              tunnel: w1318 -> [w1322]
              tunnel: w1317 -> [w1321]
              tunnel: w1316 -> [w1320]
              frame #0 {
                n835 = local write "BD 1 Frequency 1 (MHz)"(w1323) -> ()
                n836 = local write "BD 2 Frequency 1 (MHz)"(w1322) -> ()
                n837 = local write "BD 1 Frequency 2 (MHz)"(w1321) -> ()
                n838 = local write "BD 2 Frequency 2 (MHz)"(w1320) -> ()
              }
              frame #1 {
                n839 = property on="Update all trap values" class="Bool (strict)"("Val(Sgnl)"=TRUE ("Value (Signaling)")) -> ()  [unwired: 2 in, 2 out]
              }
            }
          }
        }
      }
      event "Stop All": Value Change {
        # "Stopping blue laser before shutting off program"
        n840 = event-data() -> ()  [unwired: 1 in, 5 out]
        n841 = local read "Delay (ms)"() -> (w1431:i32)
        n842 = call "serial write macro.vi"("String"="l0", "Delay (ms)"=w1431, "VISA resource name"=w1434) -> ("read buffer"=w1429:string, "error out"=w1430:errorcluster, "VISA resource name out"=w1433:refnum<visa-resource-name>)
        n843 = local write "read blue buffer"(w1429) -> ()
        n844 = local write "Blue Error Out"(w1430) -> ()
        n845 = VISA Close(VISA resource name=w1433) -> ()  [unwired: 1 in, 1 out]
        n846 = local read "Stop All"() -> (w1435:bool)
      }
      event "Sensitivity", "Offset Current Sign", "Offset Current Value", "Offset Current", "Bias Voltage", "Bias Voltage (mV)", "Filter Type", "Lowpass 3dB Point", "Highpass 3dB Point", "Filter Reset", "Invert Signal", "Gain Mode", "Send Command": Value Change {
        w1442 = 250 ("Delay (ms)")
        n847 = event-data() -> ()  [unwired: 1 in, 5 out]
        n848 = event shown="[0] \"Sensitivity\": Value Change" {
          selector: _ -> [_ _ _ _ _ _ _ _ _ _ _ _ _]
          dyn-events: _ -> [_ _ _ _ _ _ _ _ _ _ _ _ _]
          timeout: _ -> [_ _ _ _ _ _ _ _ _ _ _ _ _]
          tunnel: [w1454 w1462 w1470 w1479 w1489 w1497 w1500 w1504 w1507 w1510 w1513 w1520 "Command"] -> w1441
          tunnel: [w1449 w1456 w1466 w1473 w1483 w1493 _ _ _ _ _ w1516 _] -> w1436
          event "Sensitivity": Value Change {
            n849 = event-data() -> ()  [unwired: 1 in, 5 out]
            n850 = property on="Sensitivity" class="CmbBox"() -> ("Value"=→"Gain":string)  [unwired: 2 in, 2 out]
            n851 = Concatenate Strings("SENS ", "Sensitivity") -> (w1454:string)
            n852 = local read "Gain"() -> (w1451:string)
            n853 = Concatenate Strings("gain set at ", w1451) -> (w1449:string)
          }
          event "Offset Current Sign": Value Change {
            n854 = event-data() -> ()  [unwired: 1 in, 4 out]
            n855 = Boolean To (0,1)(Boolean="Offset Current Sign") -> (0, 1=w1465:i16)
            n856 = Select(t="positive", s="Offset Current Sign", f="negative") -> (s? t:f=w1457:string)
            n857 = Number To Decimal String(number=w1465) -> (decimal integer string=w1464:string)  [unwired: 1 in]
            n858 = Concatenate Strings("IOSN " ("string"), w1464) -> (w1462:string)
            n859 = Concatenate Strings("offset current sign ", w1457) -> (w1456:string)
          }
          event "Offset Current Value": Value Change {
            n860 = event-data() -> ()  [unwired: 1 in, 5 out]
            n861 = property on="Offset Current Value" class="CmbBox"() -> ("Value"=→"Read offset current":string)  [unwired: 2 in, 2 out]
            n862 = local read "Read offset current"() -> (w1467:string)
            n863 = Concatenate Strings("IOLV ", "Offset Current Value") -> (w1470:string)
            n864 = Concatenate Strings("offset current value ", w1467) -> (w1466:string)
          }
          event "Offset Current": Value Change {
            n865 = event-data() -> ()  [unwired: 1 in, 5 out]
            n866 = Boolean To (0,1)(Boolean="Offset Current") -> (0, 1=w1482:i16)
            n867 = Select(t="on", s="Offset Current", f="off") -> (s? t:f=w1474:string)
            n868 = Number To Decimal String(number=w1482) -> (decimal integer string=w1481:string)  [unwired: 1 in]
            n869 = Concatenate Strings("IOON " ("string"), w1481) -> (w1479:string)
            n870 = Concatenate Strings("offset current ", w1474) -> (w1473:string)
          }
          event "Bias Voltage": Value Change {
            n871 = event-data() -> ()  [unwired: 1 in, 5 out]
            n872 = Boolean To (0,1)(Boolean="Bias Voltage") -> (0, 1=w1490:i16)
            n873 = Number To Decimal String(number=w1490) -> (decimal integer string=w1491:string)  [unwired: 1 in]
            n874 = Select(t="on", s="Bias Voltage", f="off") -> (s? t:f=w1484:string)
            n875 = Concatenate Strings("BSON " ("string"), w1491) -> (w1489:string)
            n876 = Concatenate Strings("bias voltage", w1484) -> (w1483:string)
          }
          event "Bias Voltage (mV)": Value Change {
            n877 = event-data() -> ()  [unwired: 1 in, 5 out]
            n878 = Number To Decimal String(number="Bias Voltage (mV)") -> (decimal integer string=w1499:string)  [unwired: 1 in]
            n879 = Number To Fractional String(number="Bias Voltage (mV)") -> (F-format string=w1494:string)  [unwired: 3 in]
            n880 = Concatenate Strings("BSLV " ("string"), w1499) -> (w1497:string)
            n881 = Concatenate Strings("bias voltage value ", w1494) -> (w1493:string)
          }
          event "Filter Type": Value Change {
            n882 = event-data() -> ()  [unwired: 1 in, 5 out]
            n883 = Concatenate Strings("FLTT " ("string"), "Filter Type") -> (w1500:string)
          }
          event "Lowpass 3dB Point": Value Change {
            n884 = event-data() -> ()  [unwired: 1 in, 5 out]
            n885 = Concatenate Strings("LFRQ " ("string"), "Lowpass 3dB Point") -> (w1504:string)
          }
          event "Highpass 3dB Point": Value Change {
            n886 = event-data() -> ()  [unwired: 1 in, 5 out]
            n887 = Concatenate Strings("HFRQ " ("string"), "Highpass 3dB Point") -> (w1507:string)
          }
          event "Filter Reset": Value Change {
            n888 = event-data() -> ()  [unwired: 1 in, 5 out]
            n889 = Select(t="ROLD", s="Filter Reset", f="") -> (s? t:f=w1510:string)
          }
          event "Gain Mode": Value Change {
            n890 = event-data() -> ()  [unwired: 1 in, 5 out]
            n891 = Concatenate Strings("GNMD " ("string"), "Gain Mode") -> (w1513:string)
          }
          event "Invert Signal": Value Change {
            n892 = event-data() -> ()  [unwired: 1 in, 5 out]
            n893 = Boolean To (0,1)(Boolean="Invert Signal") -> (0, 1=w1523:i16)
            n894 = Number To Decimal String(number=w1523) -> (decimal integer string=w1522:string)  [unwired: 1 in]
            n895 = Concatenate Strings("INVT " ("string"), w1522) -> (w1520:string)
            n896 = Select(t="signal inverted", s="Invert Signal", f="signal not inverted") -> (s? t:f=w1516:string)
          }
          event "Send Command": Value Change {
            n897 = event-data() -> ()  [unwired: 1 in, 5 out]
          }
        }
        "Command Sent" <- w1441
        n898 = local read "Save Event Log?"() -> (w1437:bool)
        n899 = local read "Saving..."() -> (w1438:bool)
        n900 = And(x=w1437, y=w1438) -> (x .and. y?=w1439:bool)
